vi "Read_Anode_current.vi"(1 "GPIB address":string) -> (0 "Current %":dbl format="%.1f")   [LabVIEW 2010]
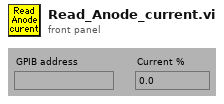
[diagram p1: front panel]
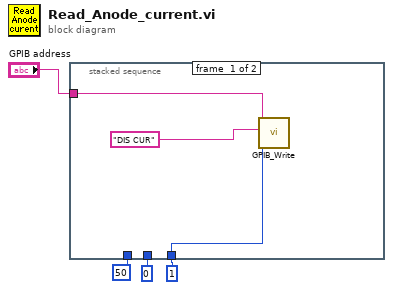
[diagram p0: block diagram]
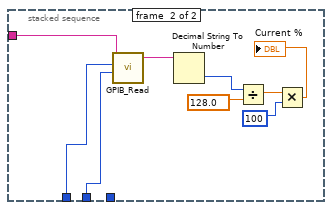
[diagram p2: hidden frame]
diagram:
  n1 = stacked-sequence {
    tunnel: "GPIB address" -> [w7 w16]
    tunnel: 1 -> [w6 _]
    tunnel: 0 -> [_ w15]
    tunnel: 50 -> [_ w14]
    frame #0 {
      n2 = call "GPIB_Write.vi"("address string"=w7, "data In"="DIS CUR", "mode (0)"=w6) -> ()  [unwired: 2 in, 2 out]
    }
    frame #1 {
      n3 = call "GPIB_Read.vi"("address string"=w16, "byte count"=w14, "mode (0)"=w15) -> ("data Out"=w13:string)  [unwired: 2 in, 2 out]
      n4 = Decimal String To Number(string=w13) -> (number=w11:i32)  [unwired: 2 in, 1 out]
      n5 = Divide(x=w11, y=128.0) -> (x/y=w9:dbl)
      n6 = Multiply(x=w9, y=100) -> (x*y=→"Current %":dbl)
    }
  }
